vi "Insert.vi"(8 "error in (no error)":errorcluster, 10 "data":dbl, 11 "List Node in":refnum<class "List.lvclass">) -> (0 "error out":errorcluster, 3 "List Node out":refnum<class "List.lvclass">)   [LabVIEW 2021, in "List.lvclass"]
doc: "本VI是为《我和LabVIEW》一书编写的示例。\n关于本书的介绍请参考网页：\nhttp://ruanqizhen.spaces.live.com/blog/cns!5852D4F797C53FB6!4310.entry"
uses:
  List.lvclass
  List.lvclass/List.ctl
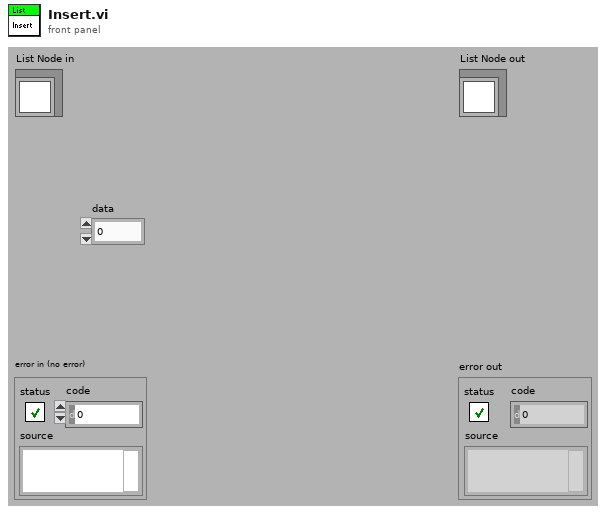
[diagram p1: front panel]
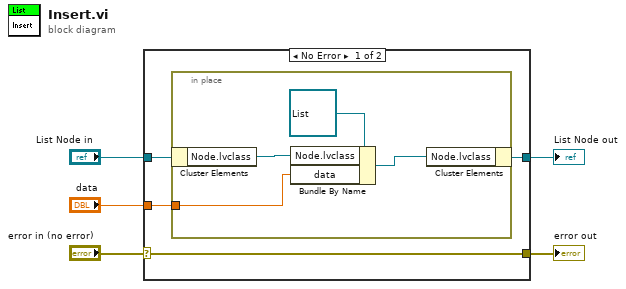
[diagram p0: block diagram]
diagram:
  n1 = case shown="No Error" "error in (no error)" {
    selector: "error in (no error)" -> [w9 w15]
    tunnel: [w9 w15] -> w4
    tunnel: [w6 w14] -> w2
    tunnel: "List Node in" -> [w8 w14]
    tunnel: "data" -> [w7 _]
    frame No Error {
      n2 = in-place {
        in-place-border: w7 -> [w10]
        n3 = in-place-cluster #1(w8) -> ("Node.lvclass"=w12:refnum<class "Node.lvclass">)
        n4 = Bundle By Name(cluster=refnum<class "List.lvclass"> refnum ("List Node in"), "Node.lvclass"=w12, "data"=w10) -> (w11:refnum<class "List.lvclass">)
        n5 = in-place-cluster #1("Node.lvclass"=w11) -> (w6:refnum<class "List.lvclass">)
      }
    }
    frame Error {
    }
  }
  "error out" <- w4
  "List Node out" <- w2
